vi "Get Connected.vi"(8 "error in (no error)":errorcluster, 11 "TCP Comm":T1) -> (0 "error out":errorcluster, 2 "Connected":bool)   [LabVIEW 2020, in "TinyTCP.lvlib"]
doc: "Returns whether the connection is currently active or not. Messages are expected to send / read while <b>Connected</b> is true.\n\nNote that due to how LabVIEW TCP works, disconnections are only detected when trying to send or receive data. This means that a TCP connection in a Connected state will continue to look as if the connection is valid until data is read or sent. To overcome this behavior, you can sent a heartbeat message as often as you want to detect a disconnection or just ensure data is continually being sent."
uses:
  TinyTCP.lvlib
  Instance.ctl
  Ref Data.ctl
  State.ctl
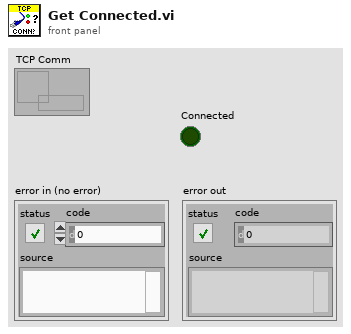
[diagram p1: front panel]
types:
  T1 = typedef "TinyTCP.lvlib/Instance.ctl" = refnum<data-value>
  T2 = typedef "TinyTCP.lvlib/State.ctl" = enum16{"Idle", "Starting", "Connecting", "Connected", "Disconnecting", "Stopped"}
  T3 = typedef "TinyTCP.lvlib/Ref Data.ctl" = cluster{"TCP":refnum<k5>, "State":T2, "Server":bool, "Host":string, "Port":u16, "Listener":refnum<k5>, "Start":bool, "Disconnect":bool, "TCP Valid":bool, "TLS Enabled":bool, "Immutable TLS":refnum<k36>, "Certificate DN":string, "local-port":u16}
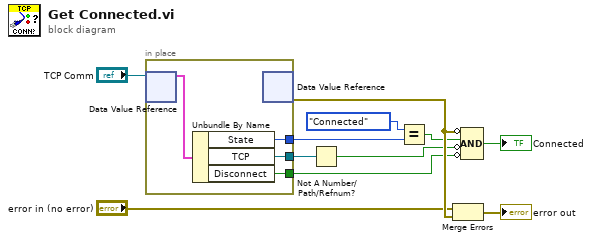
[diagram p0: block diagram]
diagram:
  n1 = in-place {
    in-place-border: [w14] -> w5
    in-place-border: [w13] -> w6
    in-place-border: [w12] -> w2
    n2 = in-place-dvr #1("TCP Comm") -> (w15:T3)  [unwired: 1 out]
    n3 = Unbundle By Name(w15) -> ("State"=w14:T2, "TCP"=w12:refnum<k5>, "Disconnect"=w13:bool)
    n4 = in-place-dvr #1() -> (w11:errorcluster)  [unwired: 1 in, 1 out]
  }
  n5 = Not A Number/Path/Refnum?(number/path/refnum=w2) -> (NaN/Path/Refnum?=w1:bool)
  n6 = Equal?(x=State."Connected", y=w5) -> (x = y?=w3:bool)
  n7 = Merge Errors("error in (no error)", w11) -> (→"error out":errorcluster)
  n8 = Compound Arithmetic op=AND(invert w11, w3, invert w1, invert w6) -> (→"Connected":bool)
